vi "Compass Facade.vi"(0 "Data In":T6, 2 "Display State In":T2={"Draw Options"={"Outer Border Color"=0, "Inner Border Color"=6316128, "Outer Gradient Color"=2565927, "Inner Gradient Color"=16860, "Compass North Pointer Color"=16711680, "Compass Pointer Color 1"=13355429, "Compass Pointer Color 2"=14934973, "Direction Pointer Color"=16765184, "Text Box Outline Color"=13355429, "Text Box Background Color"=14934973, "Scale Color"=16448250, "Text Color"=0, "Draw Gradient"=TRUE, "Draw Rose"=TRUE, "Simple Scale"=TRUE, "Draw Text"=FALSE, "Font Name"="Helvetica", "Angle Units"=enum."Degrees"}}, 3 "Container State":T5) -> (6 "Data Out":T6, 7 "Display State Out":T2={"Draw Options"={"Outer Border Color"=0, "Inner Border Color"=6316128, "Outer Gradient Color"=2565927, "Inner Gradient Color"=16860, "Compass North Pointer Color"=16711680, "Compass Pointer Color 1"=13355429, "Compass Pointer Color 2"=14934973, "Direction Pointer Color"=16765184, "Text Box Outline Color"=13355429, "Text Box Background Color"=14934973, "Scale Color"=16448250, "Text Color"=0, "Draw Gradient"=TRUE, "Draw Rose"=TRUE, "Simple Scale"=TRUE, "Draw Text"=FALSE, "Font Name"="Helvetica", "Angle Units"=enum."Degrees"}}, 8 "Action":T1)   [LabVIEW 2017, in "Compass Indicator.xctl"]
uses:
  <vilib>/robotics/Controls/Compass Indicator/Compass Indicator.xctl
  <vilib>/robotics/Controls/Compass Indicator/_Compass Indicator Support Files/Compass Data.ctl
  <vilib>/_xctls/Container State.ctl
  <vilib>/robotics/Controls/Compass Indicator/_Compass Indicator Support Files/Compass State.ctl
  <vilib>/robotics/Controls/Compass Indicator/Compass Picture/Draw Options.ctl
  <vilib>/robotics/Controls/Utilities/Angle Units.ctl
  <vilib>/_xctls/Action.ctl
  <vilib>/_xctls/XControlSupport.lvlib
  <vilib>/robotics/Controls/Utilities/NI_Robotics_Control Utilities.lvlib
  <vilib>/robotics/Controls/Compass Indicator/Compass Picture/NI_Robotics_Compass Picture.lvlib
panel:
  out "2D Picture":picture
types:
  T1 = typedef "XControlSupport.lvlib/Action.ctl" = cluster{"Data Changed?":bool, "State Changed?":bool, "Action Name":string}
  T2 = typedef "Compass Indicator.xctl/Compass State.ctl" = cluster{"Draw Options":T3}
  T3 = typedef "NI_Robotics_Compass Picture.lvlib/Draw Options.ctl" = cluster{"Outer Border Color":u32, "Inner Border Color":u32, "Outer Gradient Color":u32, "Inner Gradient Color":u32, "Compass North Pointer Color":u32, "Compass Pointer Color 1":u32, "Compass Pointer Color 2":u32, "Direction Pointer Color":u32, "Text Box Outline Color":u32, "Text Box Background Color":u32, "Scale Color":u32, "Text Color":u32, "Draw Gradient":bool, "Draw Rose":bool, "Simple Scale":bool, "Draw Text":bool, "Font Name":string, "Angle Units":T4}
  T4 = typedef "NI_Robotics_Control Utilities.lvlib/Angle Units.ctl" = enum16{"Radians", "Degrees"}
  T5 = typedef "XControlSupport.lvlib/Container State.ctl" = cluster{"Indicator?":bool, "Run Mode?":bool, " Refnum":refnum<vi>}
  T6 = typedef "Compass Indicator.xctl/Compass Data.ctl" = dbl
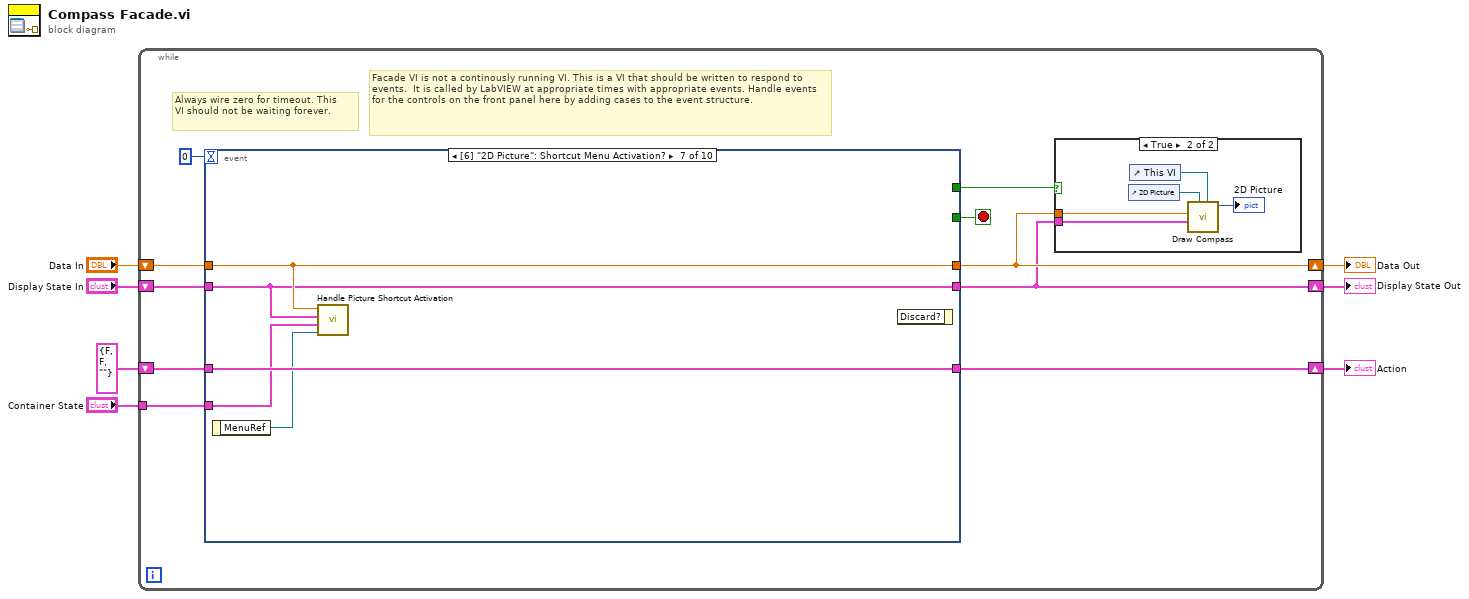
[diagram p0: block diagram]
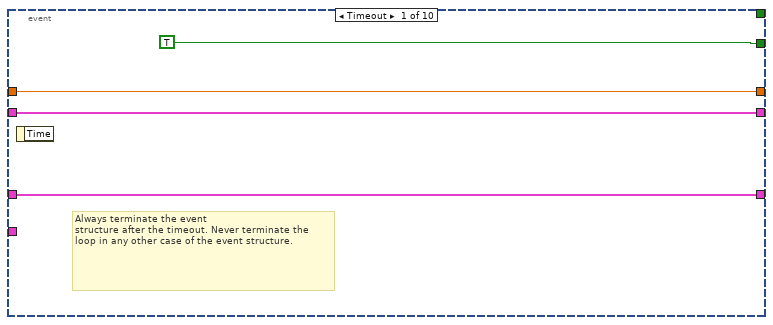
[diagram p3: hidden frame]
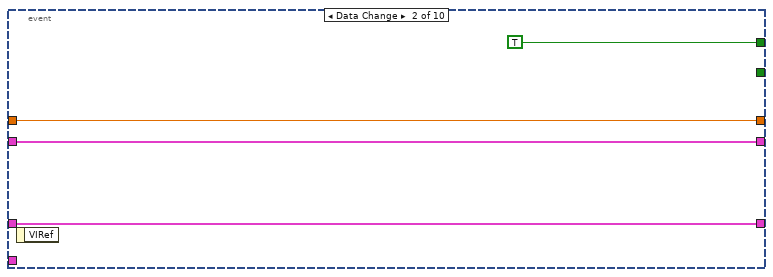
[diagram p4: hidden frame]
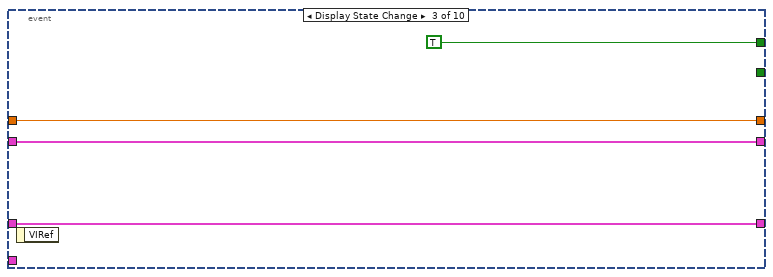
[diagram p5: hidden frame]
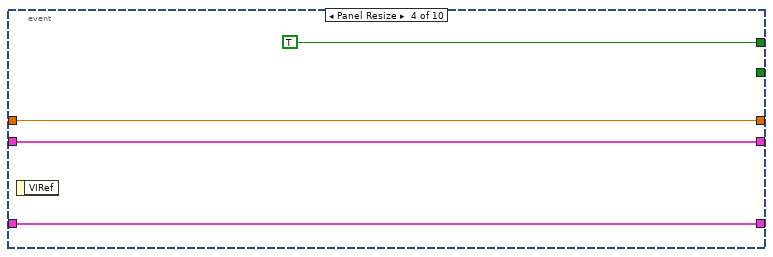
[diagram p6: hidden frame]
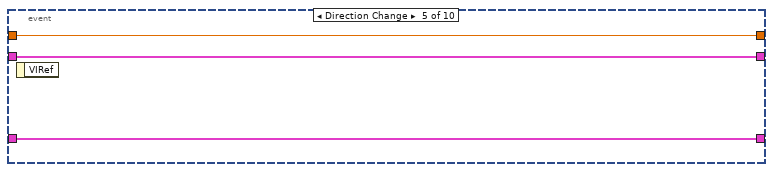
[diagram p7: hidden frame]
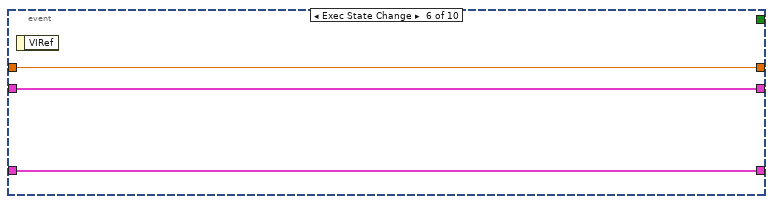
[diagram p8: hidden frame]
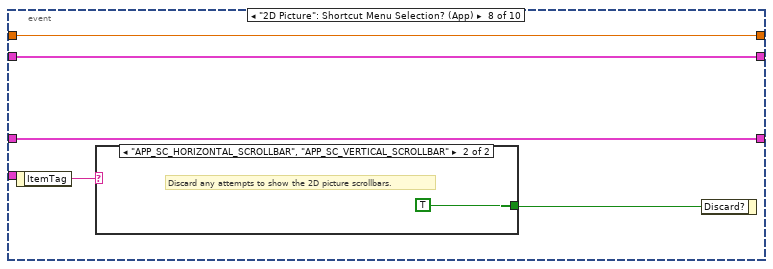
[diagram p9: hidden frame]
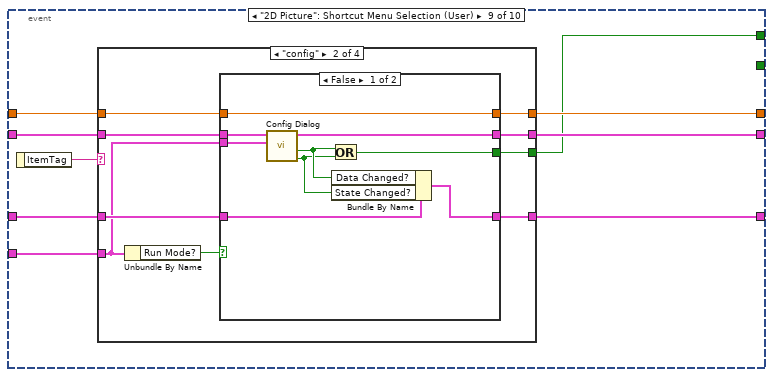
[diagram p11: hidden frame]
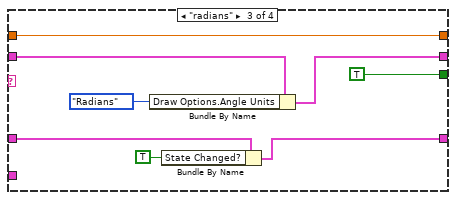
[diagram p14: hidden frame]
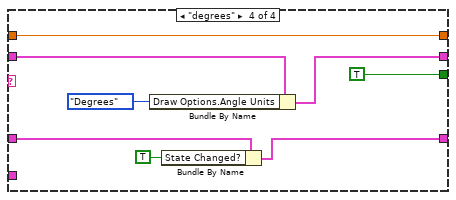
[diagram p15: hidden frame]
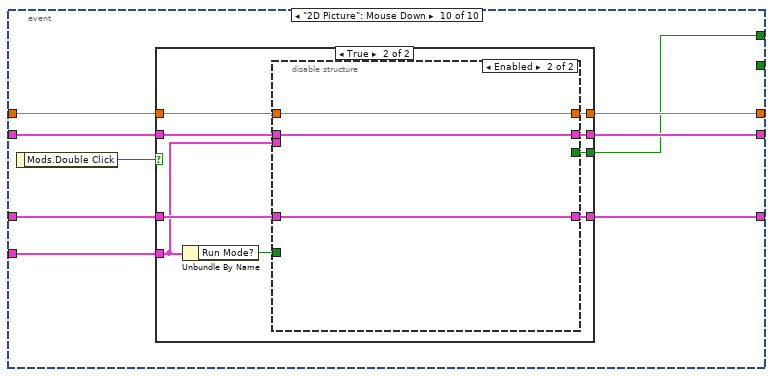
[diagram p16: hidden frame]
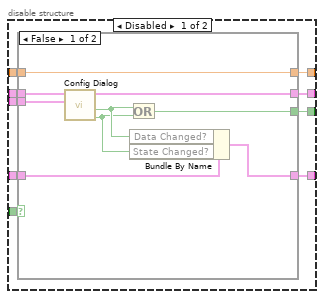
[diagram p18: hidden frame]
diagram:
  n1 = while {
    shift-right: [w9] -> w4
    shift-left: "Display State In" -> [w17]
    tunnel: "Container State" -> [w14]
    shift-right: [w10] -> w7
    shift-left: "Data In" -> [w13]
    shift-right: [w11] -> w1
    shift-left: T1 {"Data Changed?"=FALSE, "State Changed?"=FALSE, "Action Name"=""} ("Action") -> [w12]
    stop <- w16 stop-if-true
    # "Always wire zero for timeout. This\nVI should not be waiting forever."
    # "Facade VI is not a continously running VI. This is a VI that should be written to respond to events.  It is called by LabVIEW at appropriate times with appropriate events. Handle events for the controls on the front panel here by adding cases to the event structure."
    n2 = event shown="[6] \"2D Picture\": Shortcut Menu Activation?" {
      selector: _ -> [_ _ _ _ _ _ _ _ _ _]
      dyn-events: _ -> [_ _ _ _ _ _ _ _ _ _]
      timeout: 0 -> [_ _ _ _ _ _ _ _ _ _]
      tunnel: w17 -> [w25 w29 w33 w37 w41 w44 w47 w54 w62 w111]
      tunnel: [w25 w29 w33 w37 w41 w44 w47 w54 w59 w108] -> w9
      tunnel: [TRUE _ _ _ _ _ _ _ _ _] -> w16
      tunnel: w14 -> [_ _ _ _ _ _ w46 _ w57 w106]
      tunnel: w13 -> [w24 w30 w34 w38 w40 w43 w48 w53 w61 w110]
      tunnel: [w24 w30 w34 w38 w40 w43 w48 w53 w60 w109] -> w10
      tunnel: w12 -> [w23 w28 w32 w36 w39 w42 w49 w52 w63 w112]
      tunnel: [w23 w28 w32 w36 w39 w42 w49 w52 w58 w107] -> w11
      tunnel: [_ TRUE TRUE TRUE _ _ _ _ w56 w105] -> w8
      event Timeout {
        # "Always terminate the event\nstructure after the timeout. Never terminate the loop in any other case of the event structure."
        n3 = event-data() -> ()  [unwired: 1 in, 1 out]
      }
      event Data Change {
        n4 = event-data() -> ()  [unwired: 1 in, 1 out]
      }
      event Display State Change {
        n5 = event-data() -> ()  [unwired: 1 in, 1 out]
      }
      event Panel Resize {
        n6 = event-data() -> ()  [unwired: 1 in, 1 out]
      }
      event Direction Change {
        n7 = event-data() -> ()  [unwired: 1 in, 1 out]
      }
      event Exec State Change {
        n8 = event-data() -> ()  [unwired: 1 in, 1 out]
      }
      event "2D Picture": Shortcut Menu Activation? {
        n9 = event-data() -> ("MenuRef"=w45:refnum<k9>)  [unwired: 1 in]
        n10 = call <vilib>:"Handle Picture Shortcut Activation.vi"("MenuRef"=w45, "Container State"=w46, "state in"=w47, "Data"=w48) -> ()  [unwired: 8 in]
        n11 = event-data() -> ()  [unwired: 2 in, 1 out]
      }
      event "2D Picture": Shortcut Menu Selection? (App) {
        n12 = event-data() -> ("ItemTag"=w50:string)  [unwired: 1 in]
        n13 = case shown="\"APP_SC_HORIZONTAL_SCROLLBAR\", \"APP_SC_VERTICAL_SCROLLBAR\"" w50 {
          tunnel: [_ TRUE] -> w51
          frame Default {
          }
          frame "APP_SC_HORIZONTAL_SCROLLBAR", "APP_SC_VERTICAL_SCROLLBAR" {
            # "Discard any attempts to show the 2D picture scrollbars."
          }
        }
        n14 = event-data("Discard?"=w51) -> ()  [unwired: 1 in, 1 out]
      }
      event "2D Picture": Shortcut Menu Selection (User) {
        n15 = event-data() -> ("ItemTag"=w64:string)  [unwired: 1 in]
        n16 = case shown="\"config\"" w64 {
          tunnel: w63 -> [w65 w75 w90 w98]
          tunnel: w62 -> [w66 w73 w94 w102]
          tunnel: w61 -> [w67 w71 w96 w104]
          tunnel: [w67 w70 w96 w104] -> w60
          tunnel: [w66 w72 w93 w101] -> w59
          tunnel: [w65 w74 w89 w97] -> w58
          tunnel: w57 -> [_ w68 _ _]
          tunnel: [_ w69 TRUE TRUE] -> w56
          frame Default {
          }
          frame "config" {
            n17 = Unbundle By Name(w68) -> ("Run Mode?"=w76:bool)
            n18 = case shown="False" w76 {
              tunnel: w75 -> [w85 w88]
              tunnel: [w84 w88] -> w74
              tunnel: w73 -> [w78 w87]
              tunnel: [w80 w87] -> w72
              tunnel: w71 -> [w79 w86]
              tunnel: [w79 w86] -> w70
              tunnel: [w81 _] -> w69
              tunnel: w68 -> [w77 _]
              frame False {
                n19 = call <vilib>:"Config Dialog.vi"("Container State"=w77, "state in"=w78) -> ("state changed?"=w82:bool, "data changed?"=w83:bool, "state out"=w80:T2)  [unwired: 7 in]
                n20 = Or(x=w83, y=w82) -> (x .or. y?=w81:bool)
                n21 = Bundle By Name(cluster=w85, "Data Changed?"=w83, "State Changed?"=w82) -> (w84:T1)
              }
              frame True {
              }
            }
          }
          frame "radians" {
            n22 = Bundle By Name(cluster=w94, "Draw Options.Angle Units"=Angle_Units."Radians" ("Draw Options.Angle units")) -> (w93:T2)
            n23 = Bundle By Name(cluster=w90, "State Changed?"=TRUE) -> (w89:T1)
          }
          frame "degrees" {
            n24 = Bundle By Name(cluster=w102, "Draw Options.Angle Units"=Angle_Units."Degrees" ("Draw Options.Angle units")) -> (w101:T2)
            n25 = Bundle By Name(cluster=w98, "State Changed?"=TRUE) -> (w97:T1)
          }
        }
      }
      event "2D Picture": Mouse Down {
        n26 = event-data() -> ("Mods.Double Click"=w113:bool)  [unwired: 1 in]
        n27 = case shown="True" w113 {
          tunnel: w112 -> [w114 w124]
          tunnel: w111 -> [w115 w122]
          tunnel: w110 -> [w116 w120]
          tunnel: [w116 w119] -> w109
          tunnel: [w115 w121] -> w108
          tunnel: [w114 w123] -> w107
          tunnel: w106 -> [_ w117]
          tunnel: [_ w118] -> w105
          frame False {
          }
          frame True {
            n28 = Unbundle By Name(w117) -> ("Run Mode?"=w125:bool)
            n29 = disable-structure shown="Enabled" {
              disable-tunnel: w125 -> [w134 _]
              disable-tunnel: w124 -> [w133 w147]
              disable-tunnel: [w132 w147] -> w123
              disable-tunnel: w122 -> [w131 w148]
              disable-tunnel: [w130 w148] -> w121
              disable-tunnel: w120 -> [w129 w149]
              disable-tunnel: [w128 w149] -> w119
              disable-tunnel: [w127 _] -> w118
              disable-tunnel: w117 -> [w126 _]
              frame Disabled {
                n30 = case shown="False" w134 {
                  tunnel: w133 -> [w143 w146]
                  tunnel: [w142 w146] -> w132
                  tunnel: w131 -> [w137 w145]
                  tunnel: [w136 w145] -> w130
                  tunnel: w129 -> [w138 w144]
                  tunnel: [w138 w144] -> w128
                  tunnel: [w139 _] -> w127
                  tunnel: w126 -> [w135 _]
                  frame False {
                    n31 = call <vilib>:"Config Dialog.vi"("Container State"=w135, "state in"=w137) -> ("state changed?"=w140:bool, "data changed?"=w141:bool, "state out"=w136:T2)  [unwired: 7 in]
                    n32 = Or(x=w141, y=w140) -> (x .or. y?=w139:bool)
                    n33 = Bundle By Name(cluster=w143, "Data Changed?"=w141, "State Changed?"=w140) -> (w142:T1)
                  }
                  frame True {
                  }
                }
              }
              frame Enabled {
              }
            }
          }
        }
      }
    }
    n34 = case shown="True" w8 {
      tunnel: w10 -> [_ w21]
      tunnel: w9 -> [_ w20]
      frame False {
      }
      frame True {
        n35 = control-ref of="2D Picture"() -> (w19:refnum<vi>)
        n36 = control-ref of="This VI"() -> (w18:refnum<vi>)
        n37 = call <vilib>:"Draw Compass.vi"("FcdVI Refnum"=w18, "2D Picture"=w19, "State in"=w20, "Data in"=w21) -> ("picture out"=→"2D Picture":picture)  [unwired: 7 in]
      }
    }
  }
  "Display State Out" <- w4
  "Data Out" <- w7
  "Action" <- w1
